vi "Begin.vi"() -> (0 "error out":errorcluster, 1 "CameraDevRef":T1)   [LabVIEW 2011]
doc: "Called before other user functions, this VI is expected to open initial I/O refnums, load in file data, and do all program initialization. Notice that the <B>error out</B> terminal is simply used for data flow. Wiring it to other structures or subVIs ensures that this VI runs first."
uses:
  <vilib>/Rock Robotics/WPI/Camera/WPI_CameraDevRef.ctl
  <vilib>/Rock Robotics/SystemInterfaces/DIO/FPGA_DIOPWMChannel.ctl
  <vilib>/Rock Robotics/WPI/Joystick/WPI_JoystickDeviceEnum.ctl
  <vilib>/Rock Robotics/WPI/Relay/WPI_RelayDirection.ctl
  <vilib>/Rock Robotics/SystemInterfaces/DIO/FPGA_DIORelayChannel.ctl
  <vilib>/Rock Robotics/SystemInterfaces/Typedef/FPGA_TypedefDigitalModule.ctl
  <vilib>/Rock Robotics/SystemInterfaces/AI/FPGA_AIChannel.ctl
  <vilib>/Rock Robotics/WPI/MotorControl/WPI_MotorControlOpen Jaguar.vi
  <vilib>/Rock Robotics/WPI/MotorControl/WPI_MotorControlOpen Victor.vi
  Robot Global Data.vi
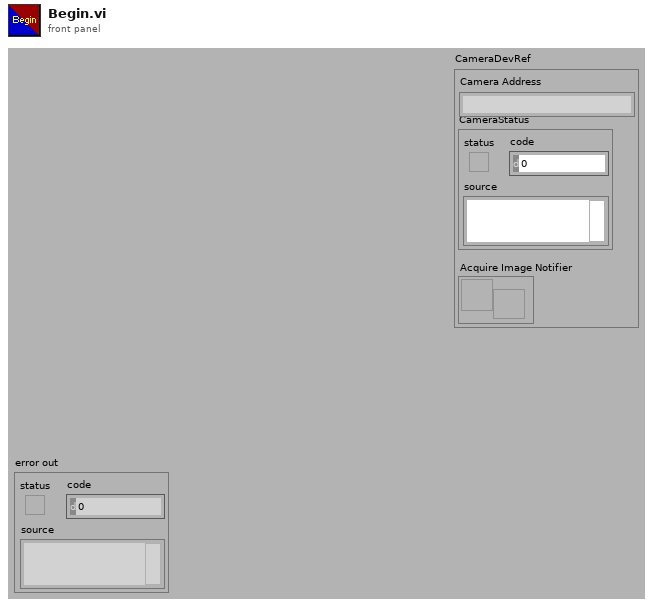
[diagram p1: front panel]
types:
  T1 = typedef "WPI_CameraDevRef.ctl" = cluster{"Camera Address":string, "CameraStatus":errorcluster, "Acquire Image Notifier":refnum<notifier>}
  T2 = typedef "FPGA_AIChannel.ctl" = enum8{"AI 1", "AI 2", "AI 3", "AI 4", "AI 5", "AI 6", "AI 7", "AI 8", "Invalid"}
  T3 = typedef "FPGA_TypedefDigitalModule.ctl" = enum16{"Digital Module 1", "Digital Module 2"}
  T4 = typedef "FPGA_DIORelayChannel.ctl" = enum8{"Relay 1", "Relay 2", "Relay 3", "Relay 4", "Relay 5", "Relay 6", "Relay 7", "Relay 8", "Invalid"}
  T5 = typedef "WPI_RelayDirection.ctl" = enum16{"Both directions", "Forward only", "Reverse only"}
  T6 = typedef "WPI_JoystickDeviceEnum.ctl" = enum16{"USB 1", "USB 2", "USB 3", "USB 4", "Kinect 1", "Kinect 2"}
  T7 = typedef "FPGA_DIOPWMChannel.ctl" = enum8{"PWM 1", "PWM 2", "PWM 3", "PWM 4", "PWM 5", "PWM 6", "PWM 7", "PWM 8", "PWM 9", "PWM 10", "Invalid"}
  T8 = typedef "WPI_CameraImageSize.ctl" = enum16{"640x480", "320x240", "160x120"}
  T9 = cluster{"fps":i32, "compression":i32, "Image Size":T8}
  T10 = typedef "WPI_CameraWhite Balance Values.ctl" = enum16{"Auto", "Fixed indoor", "Fixed outdoor 1", "Fixed outdoor 2", "Fixed fluorescent 1", "Fixed fluorescent 2", "Hold current"}
  T11 = typedef "WPI_ServoDeviceRef.ctl" = cluster{"DeviceStatus":errorcluster, "Digital Module":T3, "PWM Channel":T7, "DeadBand":T12}
  T12 = typedef "WPI_PWMDeadband.ctl" = cluster{"Name":string, "maxPositivePwm":i32, "minPositivePwm":i32, "centerPwm":i32, "maxNegativePwm":i32, "minNegativePwm":i32, "angularRange":u16}
  T13 = typedef "WPI_MotorControlDeviceRef.ctl" = cluster{"DeviceStatus":errorcluster, "Type":enum16{"PWM", "CAN"}, "PWM":cluster{"Digital Module":T3, "PWM Channel":T7, "DeadBand":T12}, "CAN":cluster{"Device Number":u8, "Control Mode":T14, "Semaphore":T15, "Max Vout":dbl}, "Invert":bool, "TransformRef":T16, "InvTransformRef":T16}
  T14 = typedef "WPI_CANJaguar_ControlMode.ctl" = enum8{"Percent VBus", "Current", "Speed", "Position", "Voltage"}
  T15 = typedef "Semaphore RefNum" = refnum<k1>
  T16 = typedef "WPI_PWMTransform_ConPane.ctl" = refnum<vi>
  T17 = typedef "WPI_CameraExposure Values.ctl" = enum16{"Auto", "Flicker-free 50 Hz", "Flicker-free 60 Hz", "Hold current"}
  T18 = typedef "WPI_AnalogChannelDevRef.ctl" = cluster{"DevStatus":errorcluster, "Analog Module":T19, "Analog Channel":T2}
  T19 = typedef "FPGA_TypedefAnalogModule.ctl" = enum16{"Analog Module 1", "Analog Module 2"}
  T20 = typedef "WPI_JoystickDevRef.ctl" = cluster{"Device":T6}
  T21 = typedef "WPI_RelayDevRef.ctl" = cluster{"DevStatus":errorcluster, "Relay Channel":T4, "Digital Module":T3, "Relay Direction":T5}
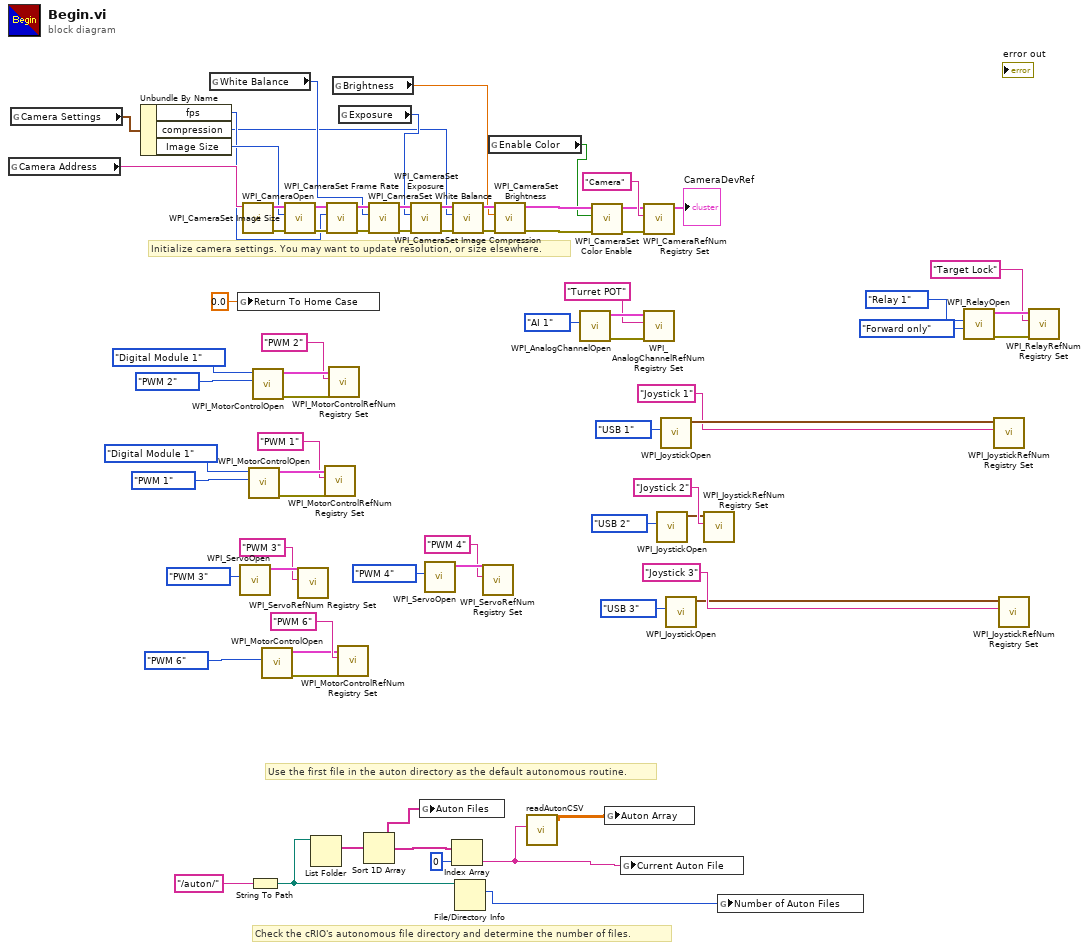
[diagram p0: block diagram]
diagram:
  # "Check the cRIO's autonomous file directory and determine the number of files."
  # "Use the first file in the auton directory as the default autonomous routine."
  # "Initialize camera settings. You may want to update resolution, or size elsewhere."
  n1 = global read "Robot Global Data.vi" "Camera Address"() -> (w61:string)
  n2 = global read "Robot Global Data.vi" "Camera Settings"() -> (w33:T9)
  n3 = Unbundle By Name(w33) -> ("fps"=w31:i32, "compression"=w28:i32, "Image Size"=w32:T8)
  n4 = global read "Robot Global Data.vi" "White Balance"() -> (w30:T10)
  n5 = global write "Robot Global Data.vi" "Return To Home Case"(0.0 ("Return To Home Case")) -> ()
  n6 = call <vilib>:"WPI_ServoOpen.vi"("PWM Channel"=FPGA_DIOPWMChannel."PWM 3") -> ("ServoDeviceRef"=w47:T11)  [unwired: 9 in, 1 out]
  n7 = call <vilib>:"WPI_CameraOpen.vi"("Camera Address"=w61) -> ("error out"=w67:errorcluster, "CameraDevRef"=w68:T1)  [unwired: 1 in, 8 out]
  n8 = call-poly <vilib>:"WPI_MotorControlOpen.vi"("PWM Channel"=FPGA_DIOPWMChannel."PWM 1", "Digital Module (Module 1)"=FPGA_TypedefDigitalModule."Digital Module 1") -> ("error out"=w53:errorcluster, "MotorControlDeviceRef"=w56:T13)  [unwired: 8 in]
  n9 = String To Path(string="/auton/") -> (path=w7:path)
  n10 = call-poly <vilib>:"WPI_MotorControlOpen.vi"("PWM Channel"=FPGA_DIOPWMChannel."PWM 2", "Digital Module (Module 1)"=FPGA_TypedefDigitalModule."Digital Module 1") -> ("error out"=w54:errorcluster, "MotorControlDeviceRef"=w59:T13)  [unwired: 8 in]
  n11 = call-poly <vilib>:"WPI_MotorControlOpen.vi"("PWM Channel"=FPGA_DIOPWMChannel."PWM 6") -> ("error out"=w42:errorcluster, "MotorControlDeviceRef"=w40:T13)  [unwired: 9 in]
  n12 = call <vilib>:"WPI_CameraSet Image Size.vi"("error in (no error)"=w67, "Image Size"=w32, "CameraDevRef"=w68) -> ("error out"=w66:errorcluster, "CameraDevRef Out"=w69:T1)  [unwired: 7 out]
  n13 = call <vilib>:"WPI_ServoRefNum Registry Set.vi"("refnum name"="PWM 3", "ServoDeviceRef"=w47) -> ()  [unwired: 8 in, 2 out]
  n14 = List Folder(path=w7) -> (filenames=w6:string[])  [unwired: 1 in, 5 out]
  n15 = call <vilib>:"WPI_MotorControlRefNum Registry Set.vi"("error in (no error)"=w53, "refnum name"="PWM 1", "MotorControlDevRef"=w56) -> ()  [unwired: 7 in, 2 out]
  n16 = call <vilib>:"WPI_CameraSet Frame Rate.vi"("error in (no error)"=w66, "Frame Rate (fps)"=w31, "CameraDevRef"=w69) -> ("error out"=w65:errorcluster, "CameraDevRef Out"=w71:T1)  [unwired: 7 out]
  n17 = call <vilib>:"WPI_MotorControlRefNum Registry Set.vi"("error in (no error)"=w54, "refnum name"="PWM 2", "MotorControlDevRef"=w59) -> ()  [unwired: 7 in, 2 out]
  n18 = global read "Robot Global Data.vi" "Brightness"() -> (w27:dbl)
  n19 = call <vilib>:"WPI_MotorControlRefNum Registry Set.vi"("error in (no error)"=w42, "refnum name"="PWM 6", "MotorControlDevRef"=w40) -> ()  [unwired: 7 in, 2 out]
  n20 = global read "Robot Global Data.vi" "Exposure"() -> (w29:T17)
  n21 = Sort 1D Array(array=w6) -> (sorted array=w1:string[])
  n22 = call <vilib>:"WPI_CameraSet White Balance.vi"("error in (no error)"=w65, "White Balance"=w30, "CameraDevRef"=w71) -> ("error out"=w64:errorcluster, "CameraDevRef Out"=w70:T1)  [unwired: 7 out]
  n23 = call <vilib>:"WPI_CameraSet Exposure.vi"("error in (no error)"=w64, "Exposure"=w29, "CameraDevRef"=w70) -> ("error out"=w63:errorcluster, "CameraDevRef Out"=w73:T1)  [unwired: 7 out]
  n24 = global write "Robot Global Data.vi" "Auton Files"(w1) -> ()
  n25 = call <vilib>:"WPI_ServoOpen.vi"("PWM Channel"=FPGA_DIOPWMChannel."PWM 4") -> ("ServoDeviceRef"=w45:T11)  [unwired: 9 in, 1 out]
  n26 = Index Array(array=w1, index=0) -> (element=w3:string)
  n27 = call <vilib>:"WPI_CameraSet Image Compression.vi"("error in (no error)"=w63, "Compression"=w28, "CameraDevRef"=w73) -> ("error out"=w62:errorcluster, "CameraDevRef Out"=w72:T1)  [unwired: 7 out]
  n28 = File/Directory Info(path=w7) -> (size=w4:i64)  [unwired: 1 in, 6 out]
  n29 = call <vilib>:"WPI_ServoRefNum Registry Set.vi"("refnum name"="PWM 4", "ServoDeviceRef"=w45) -> ()  [unwired: 8 in, 2 out]
  n30 = global read "Robot Global Data.vi" "Enable Color"() -> (w22:bool)
  n31 = call <vilib>:"WPI_CameraSet Brightness.vi"("error in (no error)"=w62, "Brightness"=w27, "CameraDevRef"=w72) -> ("error out"=w25:errorcluster, "CameraDevRef Out"=w26:T1)  [unwired: 7 out]
  n32 = call "readAutonCSV.vi"("AutonFile"=w3) -> ("AutonArray"=w2:dbl[][])  [unwired: 7 in]
  n33 = call <vilib>:"WPI_AnalogChannelOpen.vi"("Analog Channel"=FPGA_AIChannel."AI 1") -> ("error out"=w12:errorcluster, "AIDeviceRef"=w13:T18)  [unwired: 9 in]
  n34 = call <vilib>:"WPI_CameraSet Color Enable.vi"("error in (no error)"=w25, "Color Enabled"=w22, "CameraDevRef"=w26) -> ("error out"=w23:errorcluster, "CameraDevRef Out"=w24:T1)  [unwired: 7 in]
  n35 = global write "Robot Global Data.vi" "Auton Array"(w2) -> ()
  n36 = global write "Robot Global Data.vi" "Current Auton File"(w3) -> ()
  n37 = call <vilib>:"WPI_CameraRefNum Registry Set.vi"("error in (no error)"=w23, "refnum name"="Camera", "CameraDevRef"=w24) -> ("CameraDevRef"=→"CameraDevRef":T1)  [unwired: 8 out]
  n38 = call <vilib>:"WPI_AnalogChannelRefNum Registry Set.vi"("error in (no error)"=w12, "refnum name"="Turret POT", "AIDeviceRef"=w13) -> ()  [unwired: 7 in, 2 out]
  n39 = call <vilib>:"WPI_JoystickOpen.vi"("JoystickDevice"=WPI_JoystickDeviceEnum."USB 2") -> ("JoystickDevRef"=w49:T20)  [unwired: 10 in]
  n40 = call <vilib>:"WPI_JoystickOpen.vi"("JoystickDevice"=WPI_JoystickDeviceEnum."USB 1") -> ("JoystickDevRef"=w52:T20)  [unwired: 10 in]
  n41 = call <vilib>:"WPI_JoystickOpen.vi"("JoystickDevice"=WPI_JoystickDeviceEnum."USB 3") -> ("JoystickDevRef"=w37:T20)  [unwired: 10 in]
  n42 = call <vilib>:"WPI_JoystickRefNum Registry Set.vi"("refnum name"="Joystick 2", "JoystickDevRef"=w49) -> ()  [unwired: 8 in, 2 out]
  n43 = global write "Robot Global Data.vi" "Number of Auton Files"(w4) -> ()
  n44 = call <vilib>:"WPI_RelayOpen.vi"("Relay Direction"=WPI_RelayDirection."Forward only", "Relay Channel"=FPGA_DIORelayChannel."Relay 1") -> ("error out"=w19:errorcluster, "RelayDevRef"=w20:T21)  [unwired: 8 in]
  n45 = call <vilib>:"WPI_JoystickRefNum Registry Set.vi"("refnum name"="Joystick 1", "JoystickDevRef"=w52) -> ()  [unwired: 8 in, 2 out]
  n46 = call <vilib>:"WPI_JoystickRefNum Registry Set.vi"("refnum name"="Joystick 3", "JoystickDevRef"=w37) -> ()  [unwired: 8 in, 2 out]
  n47 = call <vilib>:"WPI_RelayRefNum Registry Set.vi"("error in (no error)"=w19, "refnum name"="Target Lock", "RelayDevRef"=w20) -> ()  [unwired: 7 in, 2 out]
